vi "Extension Limits Voltage Check.vi"   [LabVIEW 2013]
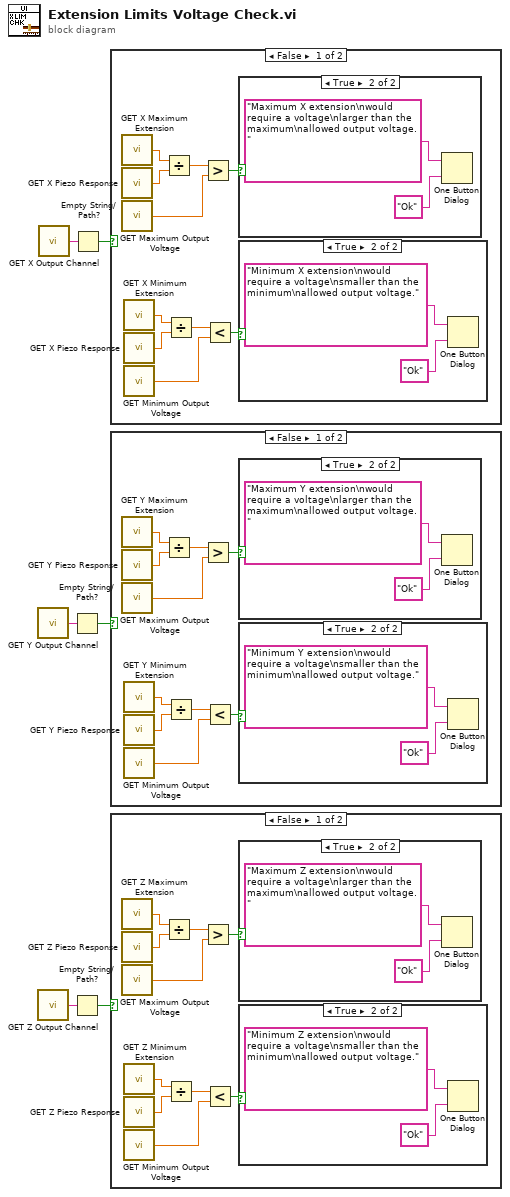
[diagram p0: block diagram]
diagram:
  n1 = call "GET Y Output Channel.vi"() -> ("Y Output Channel"=w4:string)
  n2 = call "GET Z Output Channel.vi"() -> ("Z Output Channel"=w2:string)
  n3 = call "GET X Output Channel.vi"() -> ("X Output Channel"=w6:string)
  n4 = Empty String/Path?(string/path=w4) -> (empty?=w3:bool)
  n5 = Empty String/Path?(string/path=w2) -> (empty?=w1:bool)
  n6 = Empty String/Path?(string/path=w6) -> (empty?=w5:bool)
  n7 = case shown="False" w5 {
    frame False {
      n8 = call "GET X Maximum Extension.vi"() -> ("X Maximum Extension"=w10:dbl)
      n9 = call "GET X Piezo Response.vi"() -> ("X Piezo Response"=w9:dbl)
      n10 = call "GET Maximum Output Voltage.vi"() -> ("Maximum Output Voltage"=w15:dbl)
      n11 = call "GET X Minimum Extension.vi"() -> ("X Minimum Extension"=w8:dbl)
      n12 = call "GET X Piezo Response.vi"() -> ("X Piezo Response"=w7:dbl)
      n13 = call "GET Minimum Output Voltage.vi"() -> ("Minimum Output Voltage"=w13:dbl)
      n14 = Divide(x=w10, y=w9) -> (x/y=w16:dbl)
      n15 = Divide(x=w8, y=w7) -> (x/y=w14:dbl)
      n16 = Greater?(x=w16, y=w15) -> (0:w12:bool)
      n17 = Less?(x=w14, y=w13) -> (x < y?=w11:bool)
      n18 = case shown="True" w12 {
        frame False {
        }
        frame True {
          n19 = One Button Dialog(message="Maximum X extension\nwould require a voltage\nlarger than the maximum\nallowed output voltage.", button name ("OK")="Ok") -> ()  [unwired: 1 out]
        }
      }
      n20 = case shown="True" w11 {
        frame False {
        }
        frame True {
          n21 = One Button Dialog(message="Minimum X extension\nwould require a voltage\nsmaller than the minimum\nallowed output voltage.", button name ("OK")="Ok") -> ()  [unwired: 1 out]
        }
      }
    }
    frame True {
    }
  }
  n22 = case shown="False" w3 {
    frame False {
      n23 = call "GET Y Maximum Extension.vi"() -> ("Y Maximum Extension"=w24:dbl)
      n24 = call "GET Y Piezo Response.vi"() -> ("Y Piezo Response"=w23:dbl)
      n25 = call "GET Maximum Output Voltage.vi"() -> ("Maximum Output Voltage"=w29:dbl)
      n26 = call "GET Y Minimum Extension.vi"() -> ("Y Minimum Extension"=w22:dbl)
      n27 = call "GET Y Piezo Response.vi"() -> ("Y Piezo Response"=w21:dbl)
      n28 = call "GET Minimum Output Voltage.vi"() -> ("Minimum Output Voltage"=w27:dbl)
      n29 = Divide(x=w24, y=w23) -> (x/y=w30:dbl)
      n30 = Divide(x=w22, y=w21) -> (x/y=w28:dbl)
      n31 = Greater?(x=w30, y=w29) -> (0:w26:bool)
      n32 = Less?(x=w28, y=w27) -> (x < y?=w25:bool)
      n33 = case shown="True" w26 {
        frame False {
        }
        frame True {
          n34 = One Button Dialog(message="Maximum Y extension\nwould require a voltage\nlarger than the maximum\nallowed output voltage.", button name ("OK")="Ok") -> ()  [unwired: 1 out]
        }
      }
      n35 = case shown="True" w25 {
        frame False {
        }
        frame True {
          n36 = One Button Dialog(message="Minimum Y extension\nwould require a voltage\nsmaller than the minimum\nallowed output voltage.", button name ("OK")="Ok") -> ()  [unwired: 1 out]
        }
      }
    }
    frame True {
    }
  }
  n37 = case shown="False" w1 {
    frame False {
      n38 = call "GET Z Maximum Extension.vi"() -> ("Z Maximum Extension"=w38:dbl)
      n39 = call "GET Z Piezo Response.vi"() -> ("Z Piezo Response"=w37:dbl)
      n40 = call "GET Maximum Output Voltage.vi"() -> ("Maximum Output Voltage"=w43:dbl)
      n41 = call "GET Z Minimum Extension.vi"() -> ("Z Minimum Extension"=w36:dbl)
      n42 = call "GET Z Piezo Response.vi"() -> ("Z Piezo Response"=w35:dbl)
      n43 = call "GET Minimum Output Voltage.vi"() -> ("Minimum Output Voltage"=w41:dbl)
      n44 = Divide(x=w38, y=w37) -> (x/y=w44:dbl)
      n45 = Divide(x=w36, y=w35) -> (x/y=w42:dbl)
      n46 = Greater?(x=w44, y=w43) -> (0:w40:bool)
      n47 = Less?(x=w42, y=w41) -> (x < y?=w39:bool)
      n48 = case shown="True" w40 {
        frame False {
        }
        frame True {
          n49 = One Button Dialog(message="Maximum Z extension\nwould require a voltage\nlarger than the maximum\nallowed output voltage.", button name ("OK")="Ok") -> ()  [unwired: 1 out]
        }
      }
      n50 = case shown="True" w39 {
        frame False {
        }
        frame True {
          n51 = One Button Dialog(message="Minimum Z extension\nwould require a voltage\nsmaller than the minimum\nallowed output voltage.", button name ("OK")="Ok") -> ()  [unwired: 1 out]
        }
      }
    }
    frame True {
    }
  }
